vi "Main_MultiSTSWScanning.vi"() -> ()   [LabVIEW 2014]
panel:
  out "Data Out":cluster{"Time/s":dbl[][], "Current/A":dbl[][]}
  in  "Convert To File Type":enum16{".csv", ".xlsx", ".txt"}(ring)
  out "Keithley Feedback":T1
  in  "STSW_Series":T2 {"VSleep/sec" format="%#_13g"; "VStep/V" format="%#_13g"; "VEnd/V" format="%#_13g"; "VStart/V" format="%#_13g"}
  in  "stop":bool
  in  "Channel_Series":T3 {"Switch Rate/s" format="%#_13g"}
  in  "Obj_Keithley":T4
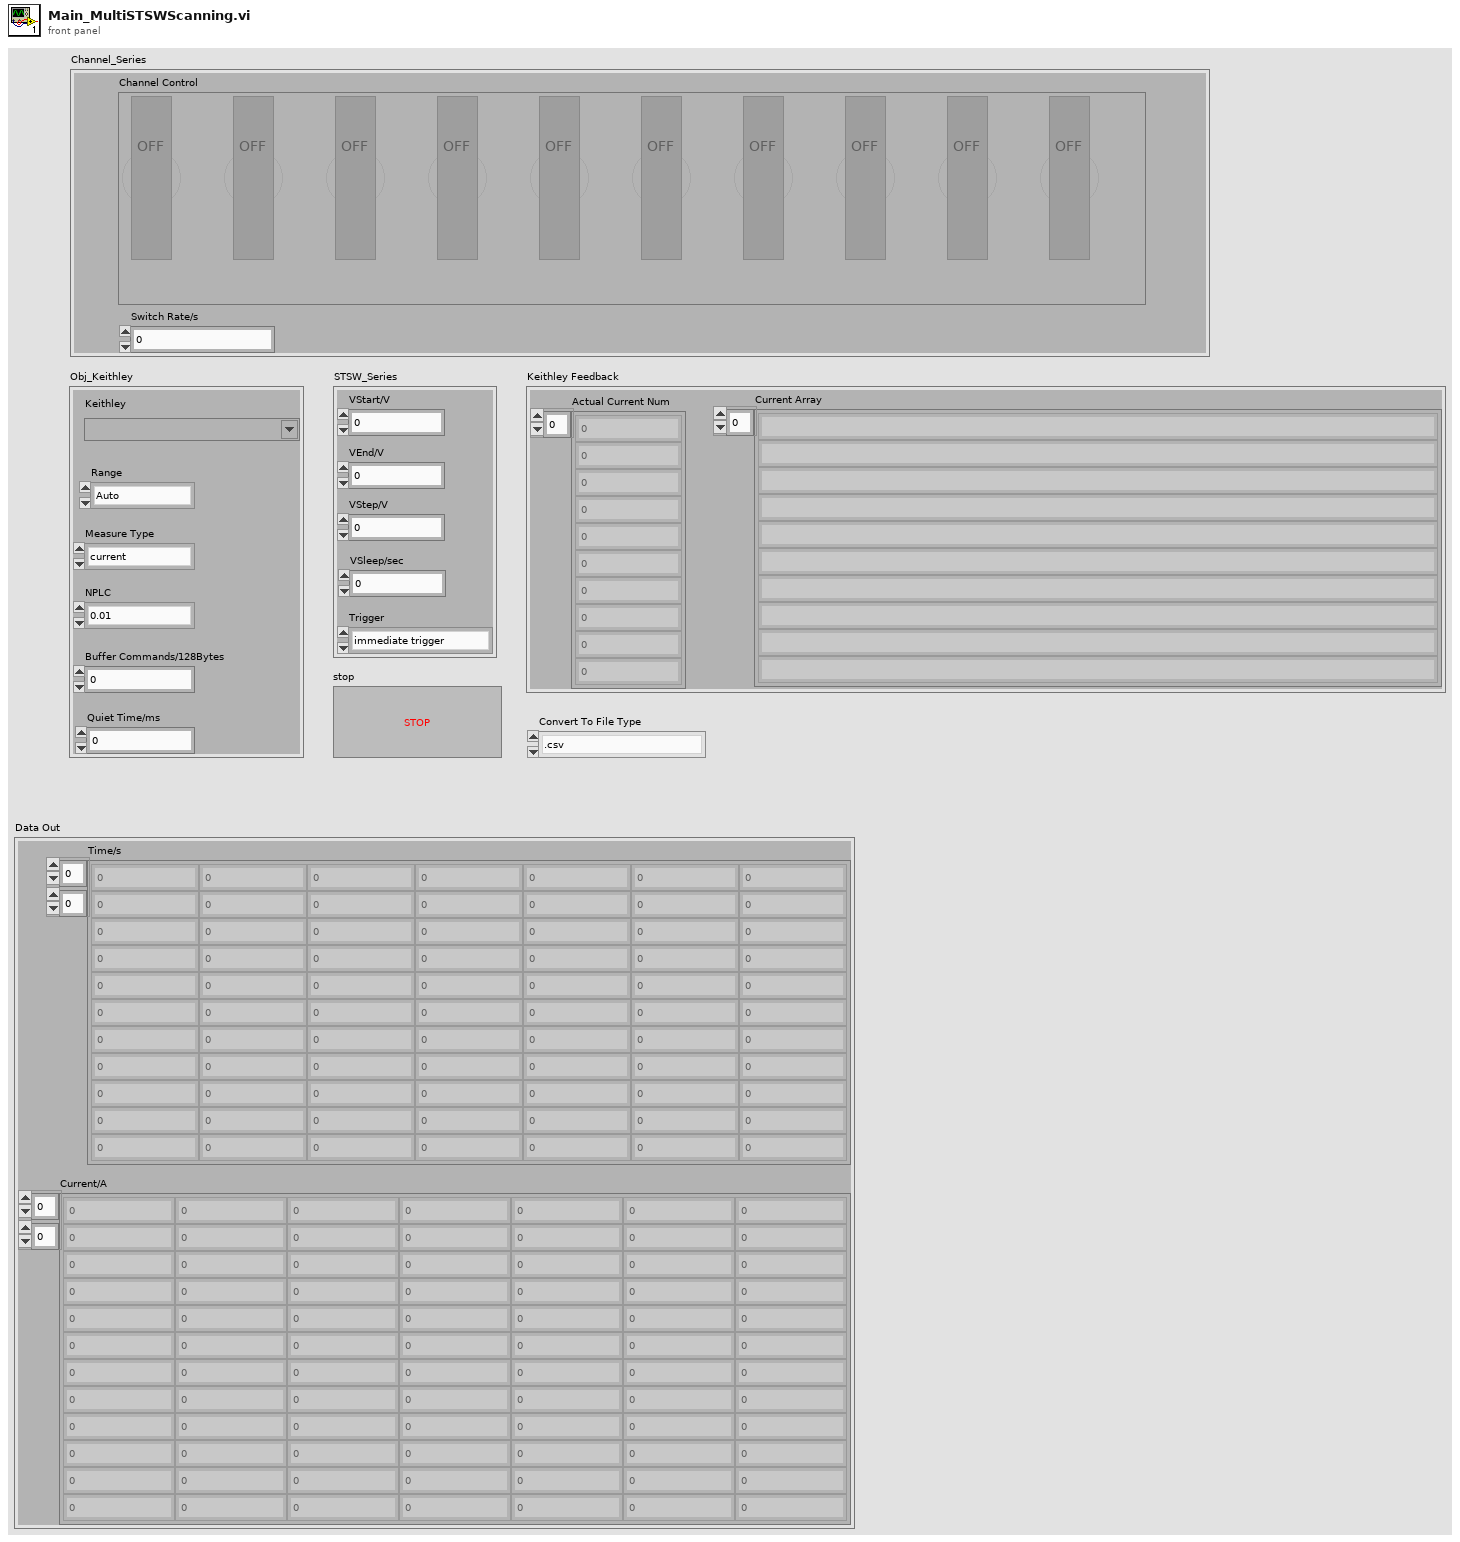
[diagram p1: front panel]
types:
  T1 = cluster{"Current Array":string[], "Actual Current Num":i32[]}
  T2 = cluster{"VStart/V":dbl, "VEnd/V":dbl, "VStep/V":dbl, "VSleep/sec":dbl, "Trigger":enum16{"immediate trigger", "delay trigger", "local trigger"}}
  T3 = cluster{"Channel Control":bool[], "Switch Rate/s":dbl}
  T4 = cluster{"Measure Type":enum16{"current", "voltage", "resistance", "charge", ""}, "NPLC":enum16{"0.01", "0.1", "1"}, "Keithley":refnum<visa-resource-name>, "Range":enum16{"Auto", "1e-1", "1e-2", "1e-3", "1e-4", "1e-5", "1e-6", "1e-7", "1e-8"}, "Buffer Commands/128Bytes":i32, "Quiet Time/ms":i32}
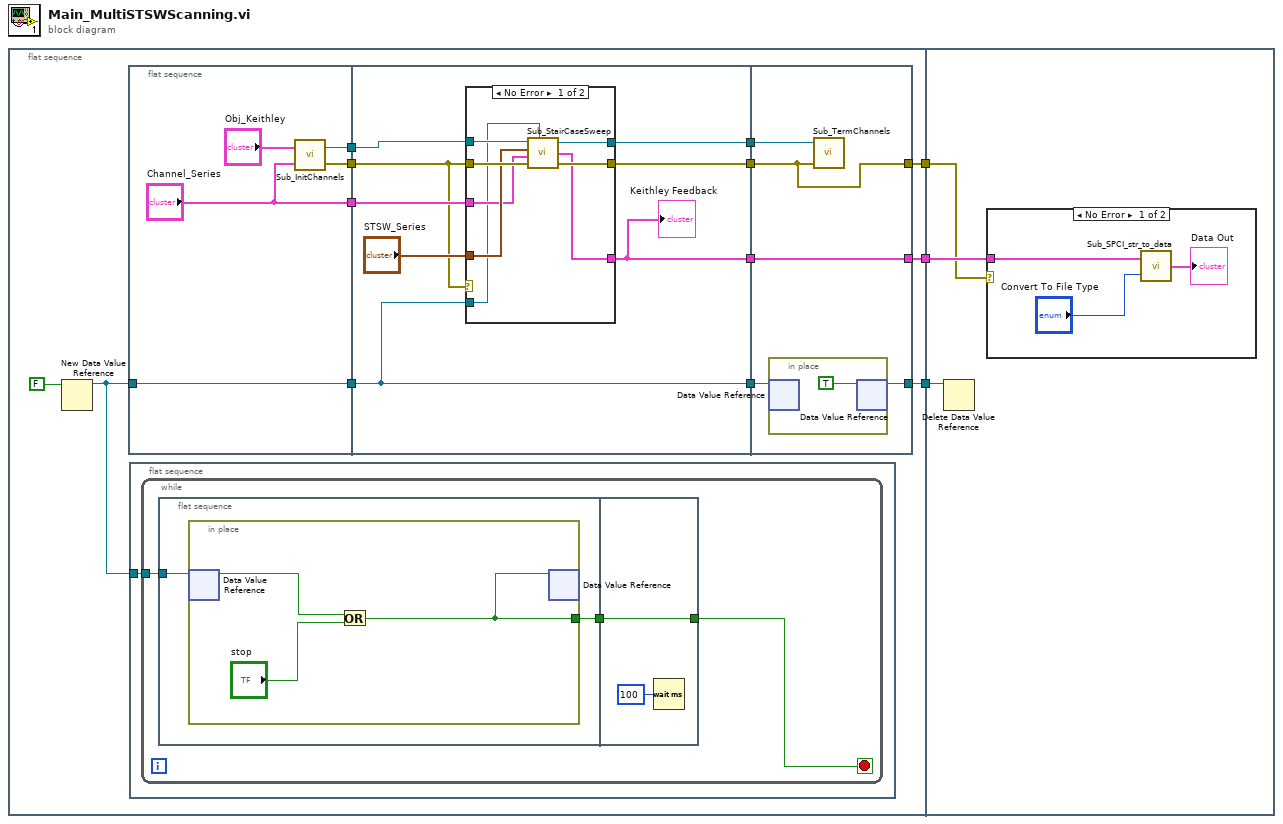
[diagram p0: block diagram]
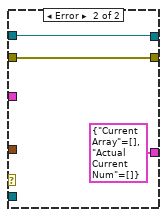
[diagram p2: hidden frame]
diagram:
  n1 = flat-sequence {
    tunnel: [w7] -> w3
    tunnel: [w5] -> w2
    tunnel: [w4] -> w1
    tunnel: w1 -> [w58]
    tunnel: w2 -> [w59]
    tunnel: w3 -> [w60]
    frame #0 {
      n2 = New Data Value Reference(data value=FALSE) -> (data value reference=w15:refnum<data-value>)  [unwired: 1 in, 1 out]
      n3 = flat-sequence {
        tunnel: w15 -> [w28]
        tunnel: [w31] -> w14
        tunnel: [w30] -> w13
        tunnel: ["Channel_Series"] -> w12
        tunnel: [w28] -> w11
        tunnel: w14 -> [w40]
        tunnel: w13 -> [w35]
        tunnel: w12 -> [w38]
        tunnel: w11 -> [w34]
        tunnel: [w37] -> w10
        tunnel: [w36] -> w9
        tunnel: [w34] -> w8
        tunnel: [w33] -> w6
        tunnel: w10 -> [w53]
        tunnel: w9 -> [w52]
        tunnel: [w55] -> w7
        tunnel: w8 -> [w56]
        tunnel: w6 -> [w54]
        tunnel: [w54] -> w5
        tunnel: [w52] -> w4
        frame #0 {
          n4 = call "Sub_InitChannels.vi"("Channel_Series"="Channel_Series", "Obj_Keithley"="Obj_Keithley") -> ("Error Out"=w30:errorcluster, "Keithley Out"=w31:refnum<visa-resource-name>)
        }
        frame #1 {
          n5 = case shown="No Error" w35 {
            tunnel: w40 -> [w48 w51]
            tunnel: w35 -> [w47 w50]
            tunnel: "STSW_Series" -> [w46 _]
            tunnel: w38 -> [w45 _]
            tunnel: [w44 w51] -> w37
            tunnel: [w43 w50] -> w36
            tunnel: [w42 T1 {"Current Array"=[], "Actual Current Num"=[]} ("Keithley Feedback")] -> w33
            tunnel: w34 -> [w41 _]
            frame No Error {
              n6 = call "Sub_StairCaseSweep.vi"("Keithley In"=w48, "STSW_Series"=w46, "Channel_Series"=w45, "Error In"=w47, "Halt Ref In"=w41) -> ("Keithley Out"=w44:refnum<visa-resource-name>, "Keithley Feedback"=w42:T1, "Error Out"=w43:errorcluster)
            }
            frame Error {
            }
          }
          "Keithley Feedback" <- w33
        }
        frame #2 {
          n7 = in-place {
            n8 = in-place-dvr #1(w56) -> ()  [unwired: 2 out]
            n9 = in-place-dvr #1(TRUE) -> (w55:refnum<data-value>)  [unwired: 1 out]
          }
          n10 = call "Sub_TermChannels.vi"("Error In"=w52, "Keithley In"=w53) -> ()
        }
      }
      n11 = flat-sequence {
        tunnel: w15 -> [w17]
        frame #0 {
          n12 = while {
            tunnel: w17 -> [w20]
            stop <- w18 stop-if-true
            n13 = flat-sequence {
              tunnel: w20 -> [w22]
              tunnel: [w21] -> w19
              tunnel: [w27] -> w18
              tunnel: w19 -> [w27]
              frame #0 {
                n14 = in-place {
                  in-place-border: [w23] -> w21
                  n15 = in-place-dvr #2(w22) -> (w25:bool)  [unwired: 1 out]
                  n16 = Or(x=w25, y="stop") -> (x .or. y?=w23:bool)
                  n17 = in-place-dvr #2(w23) -> ()  [unwired: 2 out]
                }
              }
              frame #1 {
                n18 = Wait (ms)(milliseconds to wait=u32 100) -> ()  [unwired: 1 out]
              }
            }
          }
        }
      }
    }
    frame #1 {
      n19 = Delete Data Value Reference(data value reference=w60) -> ()  [unwired: 1 in, 2 out]
      n20 = case shown="No Error" w58 {
        tunnel: w59 -> [w63 _]
        frame No Error {
          n21 = call "Sub_SPCI_str_to_data.vi"("Convert To"="Convert To File Type", "SCPI In"=w63) -> ("Data Out"=→"Data Out":cluster{"Time/s":dbl[][], "Current/A":dbl[][]})
        }
        frame Error {
        }
      }
    }
  }
